vi "FilePath.glb.vi"() -> ()   [LabVIEW 2016]
panel:
  out "modified path":path=path "C:/user/patrick/test/test/filename.000000.itx"
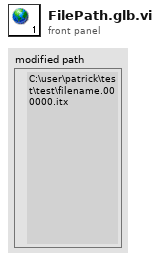
[diagram p1: front panel]
diagram:
